vi "SHCDA Specific Heat Capacity of Dry Air (KJ to Kg K).vi"(1 "Tceg":dbl[unit]) -> (0 "SHCDA":dbl[unit])   [LabVIEW 2018]
panel:
  out "SHCDA\nSpecific Heat Capacity of Dry Air\nSHCDA=0.9865+0.00010571*Tk;":dbl[unit](knob)
  out "Temprature Of Input Air\nKelvin Degree":dbl[unit](slide) scale=273.0..373.0
  out "Tk":dbl[unit]
  out "Temprature Of Input Air\nCentigrade Degree":dbl[unit](slide) scale=0.0..100.0
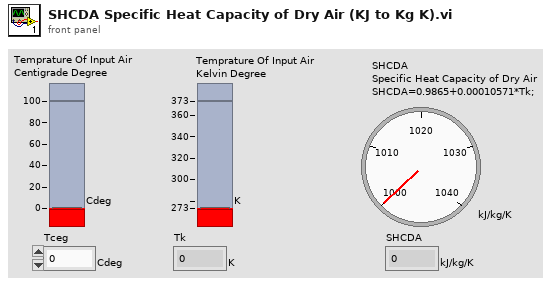
[diagram p1: front panel]
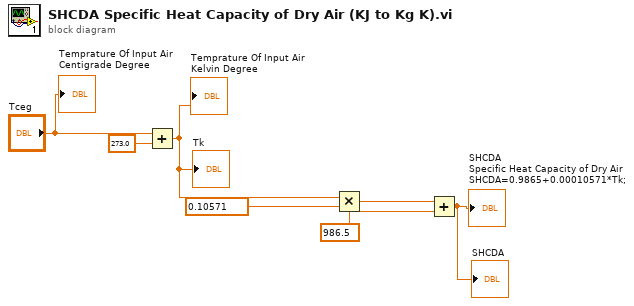
[diagram p0: block diagram]
diagram:
  n1 = Add(x="Tceg", y=dbl[unit] 273.0) -> (x+y=w1:dbl[unit])
  "Tk" <- w1
  "Temprature Of Input Air\nKelvin Degree" <- w1
  n2 = Multiply(x=w1, y=dbl[unit] 0.10571) -> (x*y=w4:dbl[unit])
  n3 = Add(x=w4, y=dbl[unit] 986.5 ("x")) -> (x+y=→"SHCDA\nSpecific Heat Capacity of Dry Air\nSHCDA=0.9865+0.00010571*Tk;" →"SHCDA":dbl[unit])
  "Temprature Of Input Air\nCentigrade Degree" <- "Tceg"
